vi "Joystick tuner.vi"() -> ()   [LabVIEW 2013]
panel:
  in  "Min":dbl
  in  "Max":dbl
  in  "Loop ID":i32=3
  in  "Joystick Z":dbl
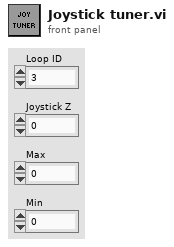
[diagram p1: front panel]
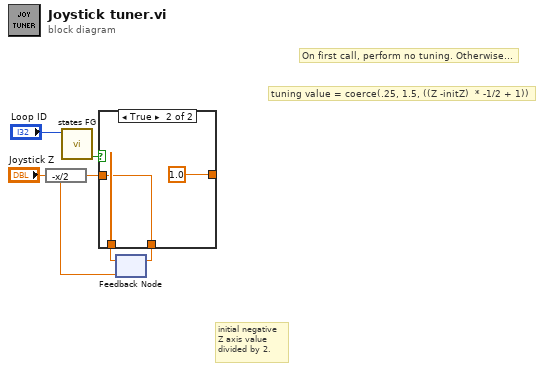
[diagram p0: block diagram]
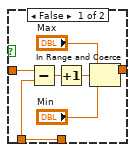
[diagram p2: hidden frame]
diagram:
  # "tuning value = coerce(.25, 1.5, ((Z -initZ)  * -1/2 + 1))"
  # "initial negative\nZ axis value\ndivided by 2."
  # "On first call, perform no tuning. Otherwise..."
  n1 = expression code="-x/2"("Joystick Z") -> (w2:dbl)
  n2 = call "states FG.vi"("Loop ID"="Loop ID") -> ("first call?"=w4:bool)  [unwired: 7 in, 3 out]
  n3 = feedback #1(w2) -> (w6:dbl)
  n4 = case shown="True" w4 {
    tunnel: w2 -> [w13 w15]
    tunnel: [w10 w15] -> w5
    tunnel: w6 -> [w10 _]
    tunnel: [w12 1.0 ("upper limit")] -> _
    frame False {
      n5 = Subtract(x=w13, y=w10) -> (x-y=w11:dbl)
      n6 = Increment(x=w11) -> (x+1=w9:dbl)
      n7 = In Range and Coerce(upper limit="Max", x=w9, lower limit="Min") -> (coerced(x)=w12:dbl)  [unwired: 1 out]
    }
    frame True {
    }
  }
  n8 = feedback-in #1(w5) -> ()
